vi "Global_InitEndSync.vi"() -> ()   [LabVIEW 2013]
panel:
  in  "Top Button":bool
  in  "Play":bool
  out "Finish":bool
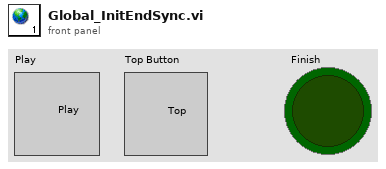
[diagram p1: front panel]
diagram:
